vi "Insert table - 3.vi"() -> ()   [LabVIEW 2015]
uses:
  <vilib>/addons/database/Connection.llb/DB Tools Open Connec (Path).vi
  <vilib>/addons/database/NI_Database_API.lvlib
panel:
  out "Average Time":dbl
  out "Time":u32
  out "Counter":i32
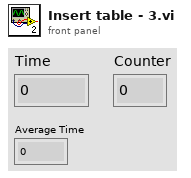
[diagram p1: front panel]
types:
  T1 = typedef "NI_Database_API.lvlib/Conn ObjectReference.ctl" = refnum<k1>
  T2 = cluster{i32, i32, i32, i32, i32, i32, i32, i32, i32, i32, i32, i32, i32, i32, i32, i32, i32, i32, i32, i32, i32, i32, i32, i32, i32, i32, i32, i32, i32, i32, i32, i32, i32, i32, i32, i32, i32, i32, i32, i32, i32, i32, i32, i32, i32, i32, i32, i32, i32, i32, i32, i32, i32, i32, i32, i32, i32, i32, i32, i32, i32, i32, i32, i32, i32, i32, i32, i32, i32, i32, i32, i32, i32, i32, i32, i32, i32, i32, i32, i32, i32, i32, i32, i32, i32, i32, i32, i32, i32, i32, i32, i32, i32, i32, i32, i32, i32, i32, i32}
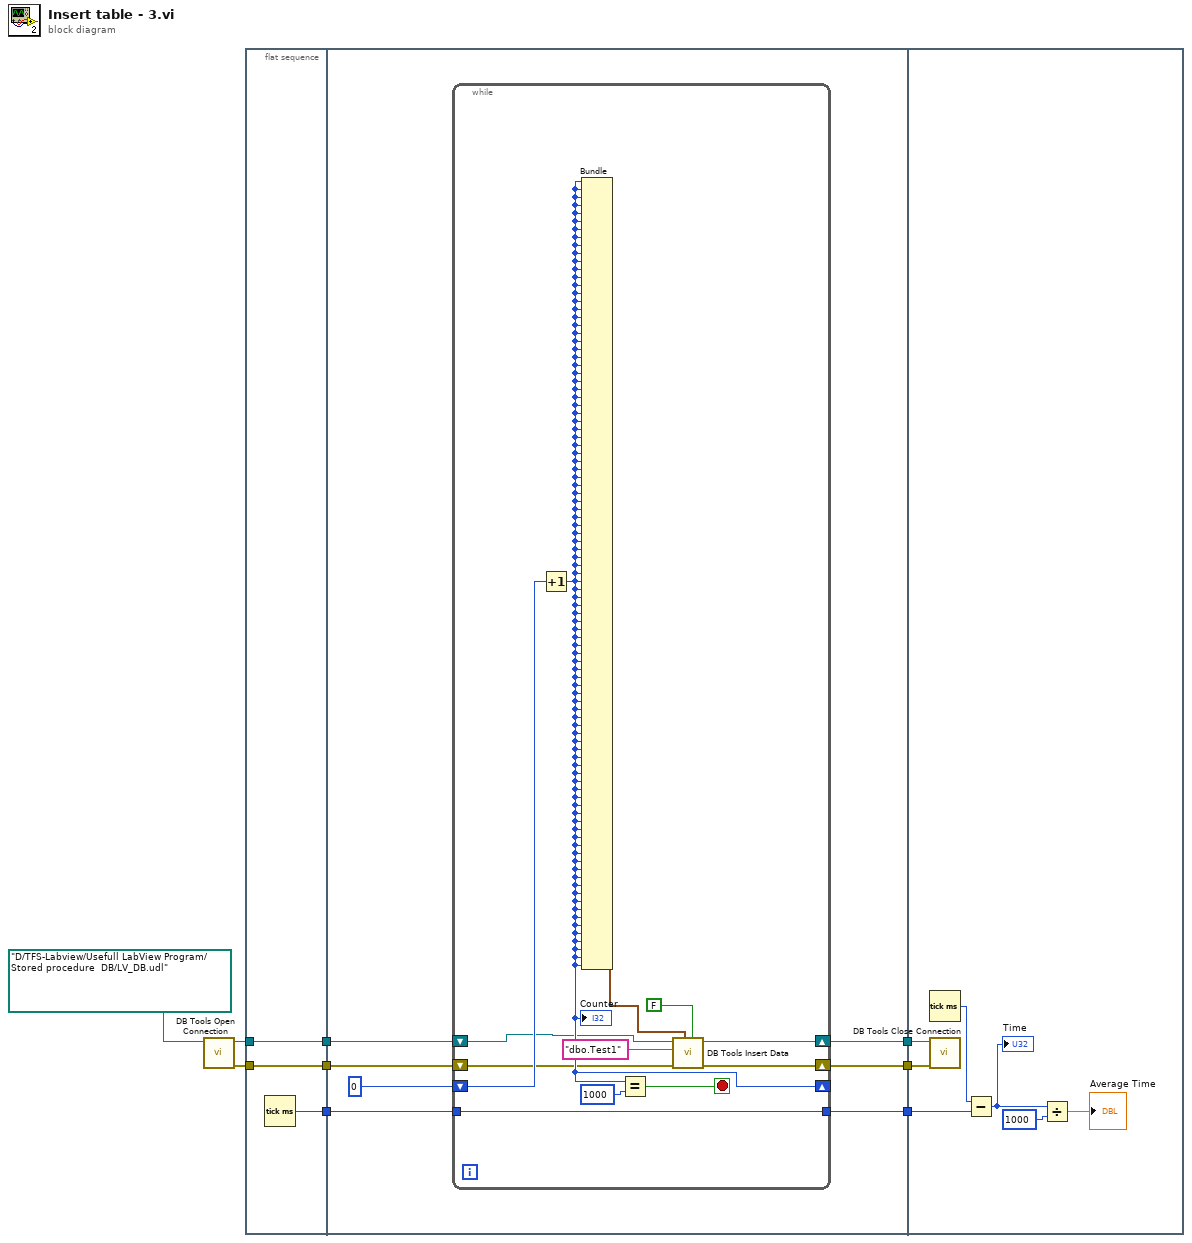
[diagram p0: block diagram]
diagram:
  n1 = call-poly <vilib>:"DB Tools Open Connection.vi"("connection information"=path "D:/TFS-Labview/Usefull LabView Program/Stored procedure  DB/LV_DB.udl") -> ("error out"=w1:errorcluster, "connection reference"=w3:T1)  [unwired: 7 in]
  n2 = flat-sequence {
    tunnel: [w12] -> w9
    tunnel: [w11] -> w8
    tunnel: w3 -> [w11]
    tunnel: [w10] -> w2
    tunnel: w1 -> [w10]
    tunnel: [w18] -> w7
    tunnel: [w16] -> w6
    tunnel: w9 -> [w17]
    tunnel: w8 -> [w15]
    tunnel: [w14] -> w5
    tunnel: w2 -> [w13]
    tunnel: w7 -> [w35]
    tunnel: w6 -> [w37]
    tunnel: w5 -> [w36]
    frame #0 {
      n3 = Tick Count (ms)() -> (millisecond timer value=w12:u32)
    }
    frame #1 {
      n4 = while {
        shift-right: [w20] -> w18
        shift-left: w13 -> [w24]
        shift-right: [w26] -> _
        shift-left: 0 -> [w31]
        tunnel: [w30] -> w16
        tunnel: w17 -> [w30]
        shift-right: [w22] -> w14
        shift-left: w15 -> [w21]
        stop <- w28 stop-if-true
        n5 = Increment(x=w31) -> (x+1=w26:i32)
        "Counter" <- w26
        n6 = Bundle(w26, w26, w26, w26, w26, w26, w26, w26, w26, w26, w26, w26, w26, w26, w26, w26, w26, w26, w26, w26, w26, w26, w26, w26, w26, w26, w26, w26, w26, w26, w26, w26, w26, w26, w26, w26, w26, w26, w26, w26, w26, w26, w26, w26, w26, w26, w26, w26, w26, w26, w26, w26, w26, w26, w26, w26, w26, w26, w26, w26, w26, w26, w26, w26, w26, w26, w26, w26, w26, w26, w26, w26, w26, w26, w26, w26, w26, w26, w26, w26, w26, w26, w26, w26, w26, w26, w26, w26, w26, w26, w26, w26, w26, w26, w26, w26, w26, w26, w26) -> (w25:T2)  [unwired: 1 in]
        n7 = Equal?(x=w26, y=1000 ("Numeric")) -> (x = y?=w28:bool)
        n8 = call <vilib>:"DB Tools Insert Data.vi"("create table? (F)"=FALSE, "data"=w25, "error in (no error)"=w24, "table"="dbo.Test1" ("SQL query"), "connection reference"=w21) -> ("error out"=w20:errorcluster, "connection reference out"=w22:T1)  [unwired: 5 in]
      }
    }
    frame #2 {
      n9 = Tick Count (ms)() -> (millisecond timer value=w38:u32)
      n10 = call <vilib>:"DB Tools Close Connection.vi"("error in (no error)"=w35, "connection reference"=w36) -> ()  [unwired: 5 in, 1 out]
      n11 = Subtract(x=w38, y=w37) -> (x-y=w34:u32)
      "Time" <- w34
      n12 = Divide(x=w34, y=u32 1000) -> (x/y=→"Average Time":dbl)
    }
  }
